vi "After Launch Init Core.vi"(8 "error in (no error)":errorcluster, 10 "DelayInitialization?":bool, 11 "BNT_ULx-MCSV-DOPWM in":refnum<class "BNT_ULx-MCSV-DOPWM.lvclass">) -> (0 "error out":errorcluster, 3 "BNT_ULx-MCSV-DOPWM out":refnum<class "BNT_ULx-MCSV-DOPWM.lvclass">)   [LabVIEW 2021, in "BNT_ULx.lvlib" / "BNT_ULx-MCSV-DOPWM.lvclass"]
doc: "Use <b>Pre Launch init.vi</b> method for sanity checks that are supposed to prevent the actor from launching if they fail. Use <B>this</B> method instead to initialize this actor when it has been activated. A corresponding high priority message will become dispatched before the <B>Actor Core.vi</b> is called.\n\n<b>Derived classed should call the parent methode first</b> and their own initialization code after.\n\nRefer also to the ongoing discussion at https://decibel.ni.com/content/message/57394#57394."
uses:
  BNT_ULx-MCSV-DOPWM.lvclass
  BNT_ULx-MCSV-DOPWM.lvclass/BNT_ULx-MCSV-DOPWM.ctl
  BNT_ULx-MCSV/BNT_ULx-MCSV.lvclass
  CSPP_Core/Classes/CSPP_ProcessVariables/CSPP_ProcessVariables.lvlib
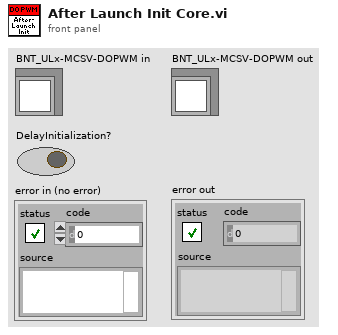
[diagram p1: front panel]
types:
  T1 = cluster{"Read Access":enum8{"Allowed", "Required", "None"}, "Write Access":enum8{"Allowed", "Required", "None"}}
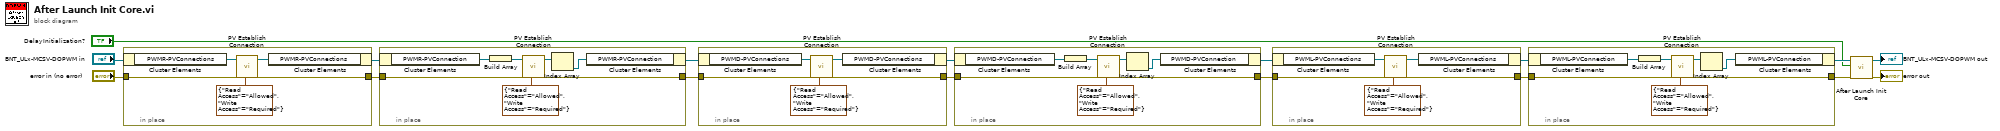
[diagram p0: block diagram]
diagram:
  n1 = in-place {
    in-place-border: [w19] -> w13
    in-place-border: "error in (no error)" -> [w22]
    n2 = in-place-cluster #1("BNT_ULx-MCSV-DOPWM in") -> ("PWMR-PVConnections"=w21:refnum<class "PVConnection.lvclass">[])
    n3 = call "PV Establish Connection.vi"("Access (R/W allowed)"=T1 {"Read Access"=enum."Allowed", "Write Access"=enum."Required"}, "Error In"=w22, "PVConnections in"=w21) -> ("Error Out"=w19:errorcluster, "PVConnections out"=w20:refnum<class "PVConnection.lvclass">[])  [unwired: 7 in]
    n4 = in-place-cluster #1("PWMR-PVConnections"=w20) -> (w12:refnum<class "BNT_ULx-MCSV-DOPWM.lvclass">)
  }
  n5 = in-place {
    in-place-border: [w26] -> w8
    in-place-border: w13 -> [w29]
    n6 = in-place-cluster #2(w12) -> ("PWMR-PVConnection"=w28:refnum<class "PVConnection.lvclass">)
    n7 = Build Array(w28) -> (w24:refnum<class "PVConnection.lvclass">[])
    n8 = call "PV Establish Connection.vi"("Access (R/W allowed)"=T1 {"Read Access"=enum."Allowed", "Write Access"=enum."Required"}, "Error In"=w29, "PVConnections in"=w24) -> ("Error Out"=w26:errorcluster, "PVConnections out"=w27:refnum<class "PVConnection.lvclass">[])  [unwired: 7 in]
    n9 = Index Array(array=w27) -> (element=w23:refnum<class "PVConnection.lvclass">)  [unwired: 1 in]
    n10 = in-place-cluster #2("PWMR-PVConnection"=w23) -> (w9:refnum<class "BNT_ULx-MCSV-DOPWM.lvclass">)
  }
  n11 = in-place {
    in-place-border: [w31] -> w10
    in-place-border: w8 -> [w34]
    n12 = in-place-cluster #3(w9) -> ("PWMD-PVConnections"=w33:refnum<class "PVConnection.lvclass">[])
    n13 = call "PV Establish Connection.vi"("Access (R/W allowed)"=T1 {"Read Access"=enum."Allowed", "Write Access"=enum."Required"}, "Error In"=w34, "PVConnections in"=w33) -> ("Error Out"=w31:errorcluster, "PVConnections out"=w32:refnum<class "PVConnection.lvclass">[])  [unwired: 7 in]
    n14 = in-place-cluster #3("PWMD-PVConnections"=w32) -> (w11:refnum<class "BNT_ULx-MCSV-DOPWM.lvclass">)
  }
  n15 = in-place {
    in-place-border: [w38] -> w5
    in-place-border: w10 -> [w41]
    n16 = in-place-cluster #4(w11) -> ("PWMD-PVConnection"=w40:refnum<class "PVConnection.lvclass">)
    n17 = Build Array(w40) -> (w36:refnum<class "PVConnection.lvclass">[])
    n18 = call "PV Establish Connection.vi"("Access (R/W allowed)"=T1 {"Read Access"=enum."Allowed", "Write Access"=enum."Required"}, "Error In"=w41, "PVConnections in"=w36) -> ("Error Out"=w38:errorcluster, "PVConnections out"=w39:refnum<class "PVConnection.lvclass">[])  [unwired: 7 in]
    n19 = Index Array(array=w39) -> (element=w35:refnum<class "PVConnection.lvclass">)  [unwired: 1 in]
    n20 = in-place-cluster #4("PWMD-PVConnection"=w35) -> (w4:refnum<class "BNT_ULx-MCSV-DOPWM.lvclass">)
  }
  n21 = in-place {
    in-place-border: [w43] -> w7
    in-place-border: w5 -> [w46]
    n22 = in-place-cluster #5(w4) -> ("PWML-PVConnections"=w45:refnum<class "PVConnection.lvclass">[])
    n23 = call "PV Establish Connection.vi"("Access (R/W allowed)"=T1 {"Read Access"=enum."Allowed", "Write Access"=enum."Required"}, "Error In"=w46, "PVConnections in"=w45) -> ("Error Out"=w43:errorcluster, "PVConnections out"=w44:refnum<class "PVConnection.lvclass">[])  [unwired: 7 in]
    n24 = in-place-cluster #5("PWML-PVConnections"=w44) -> (w6:refnum<class "BNT_ULx-MCSV-DOPWM.lvclass">)
  }
  n25 = in-place {
    in-place-border: [w50] -> w2
    in-place-border: w7 -> [w53]
    n26 = in-place-cluster #6(w6) -> ("PWML-PVConnection"=w52:refnum<class "PVConnection.lvclass">)
    n27 = Build Array(w52) -> (w48:refnum<class "PVConnection.lvclass">[])
    n28 = call "PV Establish Connection.vi"("Access (R/W allowed)"=T1 {"Read Access"=enum."Allowed", "Write Access"=enum."Required"}, "Error In"=w53, "PVConnections in"=w48) -> ("Error Out"=w50:errorcluster, "PVConnections out"=w51:refnum<class "PVConnection.lvclass">[])  [unwired: 7 in]
    n29 = Index Array(array=w51) -> (element=w47:refnum<class "PVConnection.lvclass">)  [unwired: 1 in]
    n30 = in-place-cluster #6("PWML-PVConnection"=w47) -> (w3:refnum<class "BNT_ULx-MCSV-DOPWM.lvclass">)
  }
  n31 = call-parent "After Launch Init Core.vi"("error in (no error)"=w2, "DelayInitialization?"="DelayInitialization?", "BNT_ULx-MCSV in"=w3) -> ("error out"=→"error out":errorcluster, "BNT_ULx-MCSV out"=→"BNT_ULx-MCSV-DOPWM out":refnum<class "BNT_ULx-MCSV-DOPWM.lvclass">)  [unwired: 7 in]
